vi "array-add-element-2.vi"() -> ()   [LabVIEW 2014]
panel:
  out "Array":i32[](array[numeric])
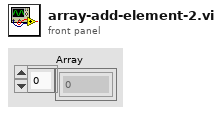
[diagram p1: front panel]
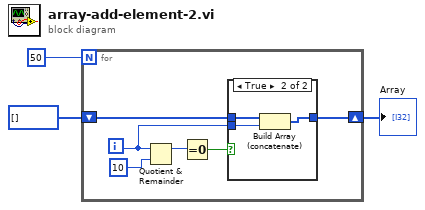
[diagram p0: block diagram]
diagram:
  n1 = for {
    N: 50 -> [_]
    shift-right: [w6] -> w2
    shift-left: i32[] [] -> [w5]
    i -> [w4]
    n2 = Quotient & Remainder(x=w4, y=10) -> (x-y*floor(x/y)=w8:i32)  [unwired: 1 out]
    n3 = Equal To 0?(x=w8) -> (x = 0?=w7:bool)
    n4 = case shown="True" w7 {
      tunnel: [w10 w13] -> w6
      tunnel: w5 -> [w10 w12]
      tunnel: w4 -> [_ w11]
      frame False {
      }
      frame True {
        n5 = Build Array (concatenate)(w12, w11) -> (w13:i32[])
      }
    }
  }
  "Array" <- w2
